vi "Set Acceleration.vi"(8 "error in (no error)":errorcluster, 10 "Array":T1[](array[typedef]), 11 "MAS in":refnum<class "MAS.lvclass">) -> (0 "error out":errorcluster, 3 "MAS out":refnum<class "MAS.lvclass">)   [LabVIEW 2022 SP3, in "MAS.lvclass"]
uses:
  MAS.lvclass
  Axis New Value.ctl
  MAS.lvclass/MAS.ctl
  iMotion Controller/iMotion Controller.lvclass
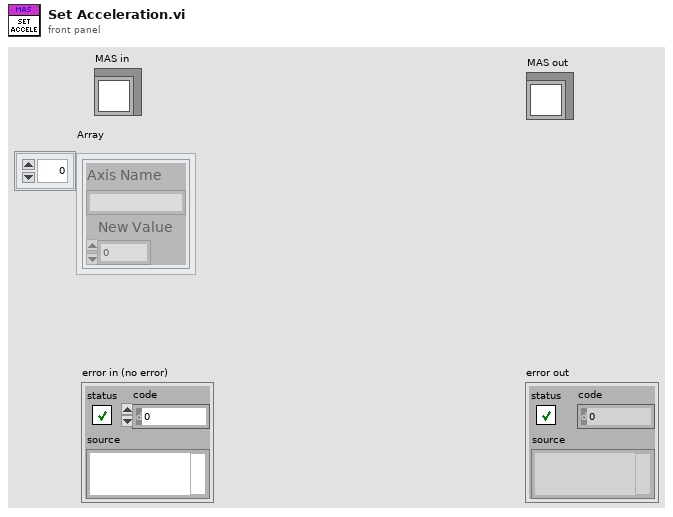
[diagram p1: front panel]
types:
  T1 = typedef "MAS.lvclass/Axis New Value.ctl" = cluster{"Axis Name":string, "New Value":dbl}
  T2 = map{string, refnum<class "iMotion Controller.lvclass">}
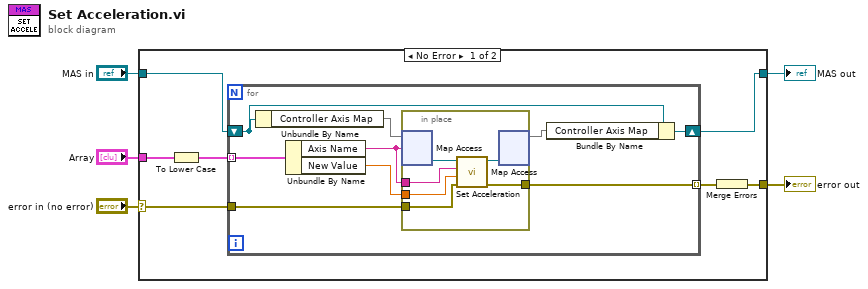
[diagram p0: block diagram]
diagram:
  n1 = case shown="No Error" "error in (no error)" {
    selector: "error in (no error)" -> [w9 w29]
    tunnel: [w7 w29] -> w4
    tunnel: [w10 w28] -> w2
    tunnel: "MAS in" -> [w11 w28]
    tunnel: "Array" -> [w12 _]
    frame No Error {
      n2 = To Lower Case(string=w12) -> (all lower case string=w6:T1[])
      n3 = for {
        tunnel: w6 -> [w20] mode=indexing
        shift-right: [w15] -> w10
        shift-left: w11 -> [w17]
        tunnel: w9 -> [w14]
        tunnel: [w13] -> w8 mode=indexing
        n4 = Unbundle By Name(w17) -> ("Controller Axis Map"=w21:T2)
        n5 = Unbundle By Name(w20) -> ("Axis Name"=w19:string, "New Value"=w18:dbl)
        n6 = in-place {
          in-place-border: w19 -> [w26]
          in-place-border: w18 -> [w25]
          in-place-border: w14 -> [w23]
          in-place-border: [w22] -> w13
          n7 = in-place-map #1(w21, w19) -> (w27:refnum<class "iMotion Controller.lvclass">)  [unwired: 1 in, 1 out]
          n8 = call-dynamic "Set Acceleration.vi"("error in (no error)"=w23, "Acceleration"=w25, "Axis Name"=w26, "iMotion Controller in"=w27) -> ("error out"=w22:errorcluster, "iMotion Controller out"=w24:refnum<class "iMotion Controller.lvclass">)  [unwired: 6 in]
          n9 = in-place-map #1(w24) -> (w16:T2)  [unwired: 1 in, 2 out]
        }
        n10 = Bundle By Name(cluster=w17, "Controller Axis Map"=w16) -> (w15:refnum<class "MAS.lvclass">)
      }
      n11 = Merge Errors(w8) -> (w7:errorcluster)
    }
    frame Error {
    }
  }
  "error out" <- w4
  "MAS out" <- w2
